vi "Check Loop Error.vi"(6 "错误时退出？ (F)":bool, 9 "忽略错误":i32[](array[numeric]), 10 "待处理的错误":cluster{"状态":bool, "代码":i32, "源":string}, 11 "消息队列":refnum<queue>) -> (2 "出错？":bool, 3 "消息队列副本":refnum<queue>)   [LabVIEW 2025]
doc: "检查“待处理消息”的代码是否与“忽略错误”数组中的任意一项匹配。如存在匹配，则不做处理。如不存在匹配，则向“消息处理循环”发送包含错误数据的Error消息，以便对错误进一步处理。如“错误时退出？”的输入为真，则向消息处理循环发送“退出”消息。"
uses:
  Message Queue/Message Cluster.ctl
  Message Queue/Enqueue Message (Single).vi
  Message Queue/Message Queue.lvlib
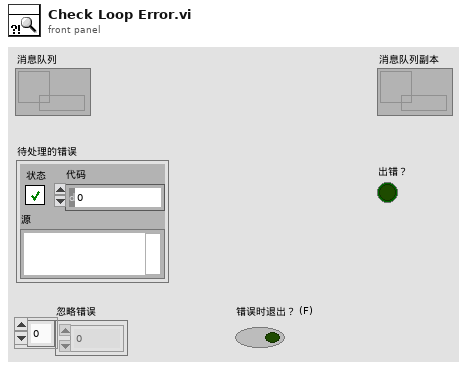
[diagram p1: front panel]
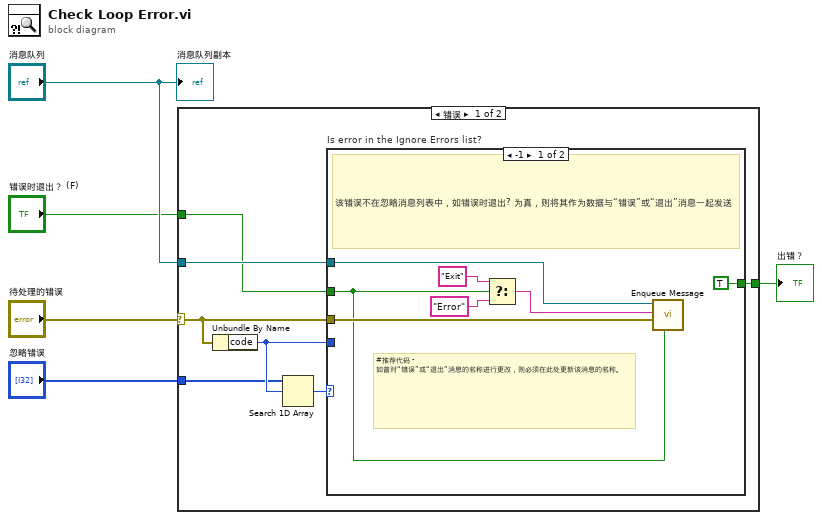
[diagram p0: block diagram]
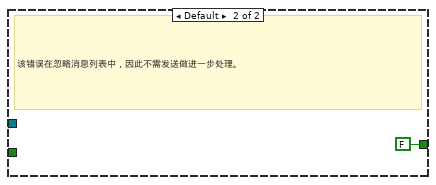
[diagram p2: hidden frame]
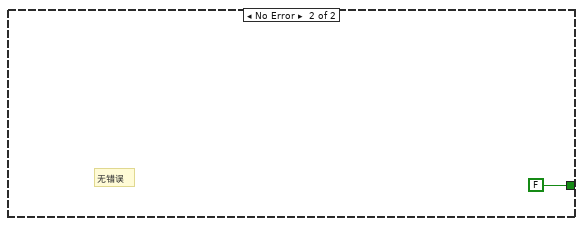
[diagram p3: hidden frame]
diagram:
  n1 = case shown="错误" "待处理的错误" {
    selector: "待处理的错误" -> [w9 _]
    tunnel: "消息队列" -> [w12 _]
    tunnel: "忽略错误" -> [w8 _]
    tunnel: [w7 FALSE] -> w2
    tunnel: "错误时退出？ (F)" -> [w6 _]
    frame Error {
      n2 = Unbundle By Name(w9) -> ("code"=w10:i32)
      n3 = Search 1D Array(1D array=w8, element=w10) -> (index of element=w11:i32)  [unwired: 1 in]
      n4 = case "Is error in the Ignore Errors list?" shown="-1" w11 {
        tunnel: w9 -> [w17 _]
        tunnel: w12 -> [w19 _]
        tunnel: w10 -> [_ _]
        tunnel: [TRUE FALSE] -> w7
        tunnel: w6 -> [w16 _]
        frame -1 {
          # "#推荐代码 - 如曾对“错误”或“退出”消息的名称进行更改，则必须在此处更新该消息的名称。"
          # "该错误不在忽略消息列表中，如错误时退出? 为真，则将其作为数据与“错误”或“退出”消息一起发送"
          n5 = Select(t="Exit" ("Message"), s=w16, f="Error" ("Message")) -> (s? t:f=w15:string)
          n6 = call-poly "Enqueue Message.vi"("优先消息？ (F)"=w16, "消息数据"=w17, "消息"=w15, "消息队列"=w19) -> ()  [unwired: 6 in, 2 out]
        }
        frame Default {
          # "该错误在忽略消息列表中，因此不需发送做进一步处理。"
        }
      }
    }
    frame No Error {
      # "无错误"
    }
  }
  "出错？" <- w2
  "消息队列副本" <- "消息队列"
